vi "KillProcess.vi"() -> ()   [LabVIEW 2013]
panel:
  in  "COMIn":refnum<visa-resource-name>
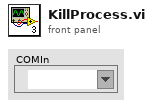
[diagram p1: front panel]
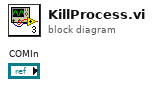
[diagram p0: block diagram]
diagram:
